vi "Destructor.vi"(8 "ErrorIn":errorcluster, 11 "Car:Car in":refnum<class "Car.lvclass">) -> (0 "ErrorOut":errorcluster, 3 "Car:Car out":refnum<class "Car.lvclass">)   [LabVIEW 2021, in "Car.lvlib" / "Car.lvclass"]
uses:
  Car.lvclass
  Car.lvclass/Car.ctl
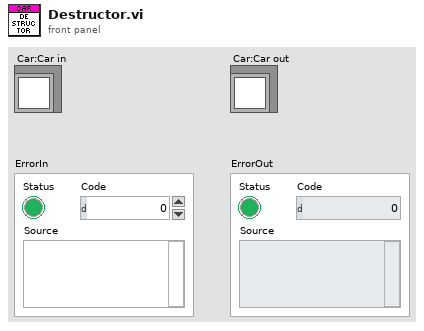
[diagram p1: front panel]
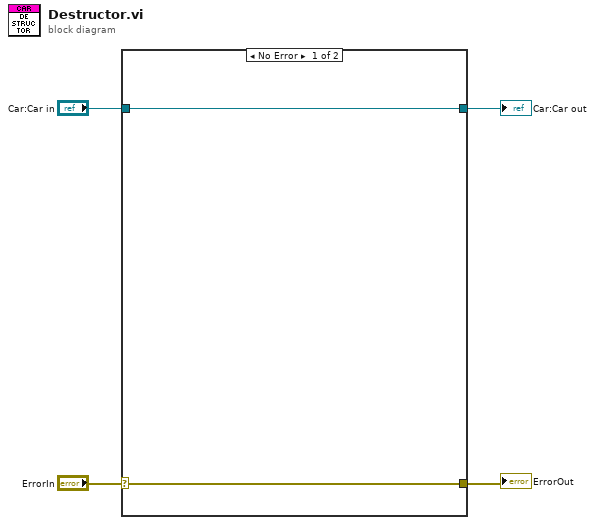
[diagram p0: block diagram]
diagram:
  n1 = case shown="No Error" "ErrorIn" {
    selector: "ErrorIn" -> [w5 w8]
    tunnel: [w5 w8] -> w3
    tunnel: [w6 w7] -> w1
    tunnel: "Car:Car in" -> [w6 w7]
    frame No Error {
    }
    frame Error {
    }
  }
  "ErrorOut" <- w3
  "Car:Car out" <- w1
